vi "Poll_tracker_171213.vi"(0 "VISA resource name":refnum<visa-resource-name>="ASRL3::INSTR", 5 "error in (no error)":errorcluster) -> (12 "read buffer":string, 14 "VISA resource name out":refnum<visa-resource-name>, 15 "Binary mode status":string, 16 "Coordinate mode status":string, 17 "Matrix mode status":string, 18 "FPS status":i32, 19 "error out":errorcluster)   [LabVIEW 2016]
panel:
  out "Poll records":u32
  out "FPS target index":i32
  out "Matrix mode index":i32
  out "Coordinate mode index":i32
  out "Binary mode index":i32
  out "Array of tokens":string[](array[string])
  out "token index":i32
  out "Serial Settings:Number of Bytes at Serial Port":u32
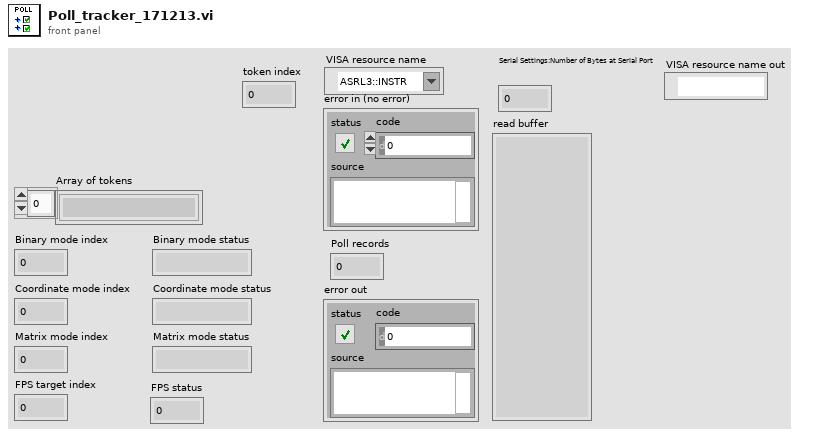
[diagram p1: front panel]
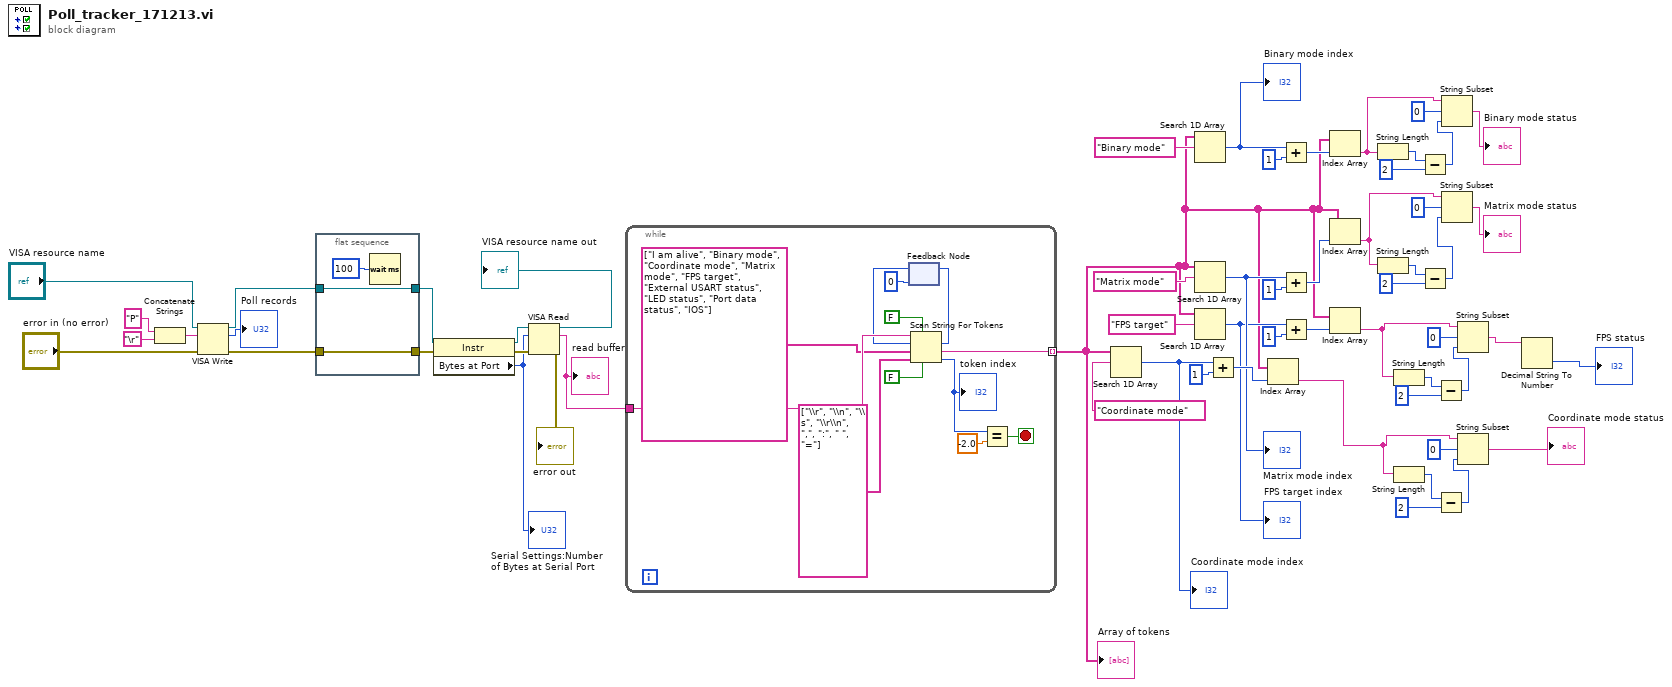
[diagram p0: block diagram]
diagram:
  n1 = Concatenate Strings("P" ("write buffer"), "\r") -> (w56:string)
  n2 = VISA Write(VISA resource name="VISA resource name", write buffer=w56, error in (no error)="error in (no error)") -> (VISA resource name out=w30:refnum<visa-resource-name>, return count=→"Poll records":u32, error out=w28:errorcluster)
  n3 = flat-sequence {
    tunnel: [w60] -> w31
    tunnel: w30 -> [w60]
    tunnel: [w59] -> w29
    tunnel: w28 -> [w59]
    frame #0 {
      n4 = Wait (ms)(milliseconds to wait=u32 100) -> ()  [unwired: 1 out]
    }
  }
  n5 = property class="Instr"(reference=w31, error in=w29) -> (reference out=w54:refnum<visa-resource-name>, error out=w53:errorcluster, "Bytes at Port"=w52:u32)
  "Serial Settings:Number of Bytes at Serial Port" <- w52
  n6 = VISA Read(VISA resource name=w54, byte count=w52, error in (no error)=w53) -> (VISA resource name out=→"VISA resource name out":refnum<visa-resource-name>, read buffer=w51:string, error out=→"error out":errorcluster)  [unwired: 1 out]
  "read buffer" <- w51
  n7 = while {
    tunnel: w51 -> [w73]
    tunnel: [w62] -> w34 mode=indexing
    stop <- w69 stop-if-true
    n8 = feedback #1(0 ("offset past token")) -> (w70:i32)
    n9 = Scan String For Tokens(4:FALSE ("use cached delim/oper data? (F)"), 5:FALSE ("allow empty tokens? (F)"), 6:string[] ["\\r", "\\n", "\\s", "\\r\\n", ",", ":", " ", "="] ("delimiters"), 7:string[] ["I am alive", "Binary mode", "Coordinate mode", "Matrix mode", "FPS target", "External USART status", "LED status", "Port data status", "IOS"] ("Tokens"), 8:w70, 9:w73) -> (0:w67:i32, 1:w62:string, 2:w71:i32)  [unwired: 1 out]
    "token index" <- w67
    n10 = feedback-in #1(w71) -> ()
    n11 = Equal?(x=w67, y=-2.0) -> (x = y?=w69:bool)
  }
  "Array of tokens" <- w34
  n12 = Search 1D Array(1D array=w34, element="Coordinate mode") -> (index of element=w44:i32)  [unwired: 1 in]
  "Coordinate mode index" <- w44
  n13 = Search 1D Array(1D array=w34, element="Binary mode") -> (index of element=w48:i32)  [unwired: 1 in]
  "Binary mode index" <- w48
  n14 = Search 1D Array(1D array=w34, element="Matrix mode") -> (index of element=w40:i32)  [unwired: 1 in]
  "Matrix mode index" <- w40
  n15 = Search 1D Array(1D array=w34, element="FPS target") -> (index of element=w36:i32)  [unwired: 1 in]
  "FPS target index" <- w36
  n16 = Add(x=w44, y=1) -> (x+y=w45:i32)
  n17 = Index Array(array=w34, index=w45) -> (element=w1:string)
  n18 = Add(x=w48, y=1) -> (x+y=w49:i32)
  n19 = Add(x=w40, y=1) -> (x+y=w41:i32)
  n20 = Add(x=w36, y=1) -> (x+y=w37:i32)
  n21 = Index Array(array=w34, index=w49) -> (element=w24:string)
  n22 = Index Array(array=w34, index=w41) -> (element=w3:string)
  n23 = Index Array(array=w34, index=w37) -> (element=w2:string)
  n24 = String Length(string=w24) -> (length=w23:i32)
  n25 = String Length(string=w3) -> (length=w18:i32)
  n26 = String Length(string=w2) -> (length=w13:i32)
  n27 = String Length(string=w1) -> (length=w7:i32)
  n28 = Subtract(x=w23, y=2) -> (x-y=w21:i32)
  n29 = Subtract(x=w18, y=2) -> (x-y=w16:i32)
  n30 = Subtract(x=w13, y=2) -> (x-y=w11:i32)
  n31 = Subtract(x=w7, y=2) -> (x-y=w5:i32)
  n32 = String Subset(string=w24, offset (0)=0, length (rest)=w21) -> (substring=→"Binary mode status":string)
  n33 = String Subset(string=w3, offset (0)=0, length (rest)=w16) -> (substring=→"Matrix mode status":string)
  n34 = String Subset(string=w2, offset (0)=0, length (rest)=w11) -> (substring=w10:string)
  n35 = String Subset(string=w1, offset (0)=0, length (rest)=w5) -> (substring=→"Coordinate mode status":string)
  n36 = Decimal String To Number(string=w10) -> (number=→"FPS status":i32)  [unwired: 2 in, 1 out]
